vi "Stop Core.vi"(10 "final error code":i32, 11 "SinglePhotonInterferenceUI in":refnum<class "SinglePhotonInterferenceUI.lvclass">) -> (3 "SinglePhotonInterferenceUI out":refnum<class "SinglePhotonInterferenceUI.lvclass">)   [LabVIEW 2023, in "SinglePhotonInterferenceUI.lvlib" / "SinglePhotonInterferenceUI.lvclass"]
doc: "(<B>Filename</B>: Actor Framework.lvlib:Actor.lvclass:Stop Core.vi)\n\nDefines what the actor does before it stops. Use the <B>final error code</B> input to determine whether the actor shut down in response to an error.\n\nBy default, this method passes the Stop message along to all auto-stop nested actors. A descendant class may override this method to define additional behavior, such as shutting down any processes the actor initiated in its override of the Actor Core method."
uses:
  SinglePhotonInterferenceUI.lvclass
  <vilib>/ActorFramework/Actor/Actor.lvclass
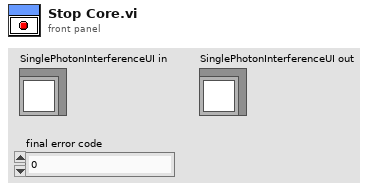
[diagram p1: front panel]
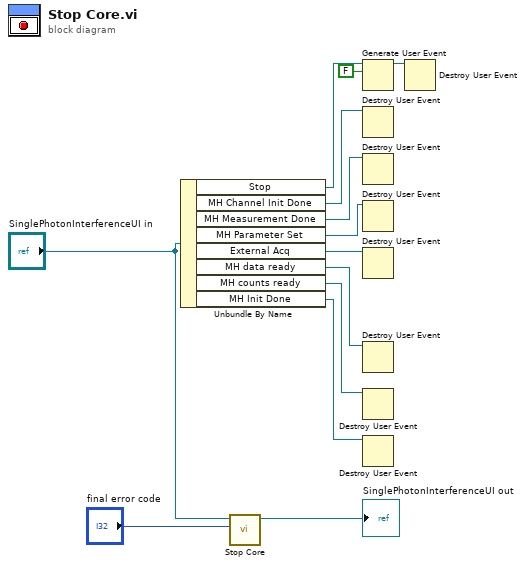
[diagram p0: block diagram]
diagram:
  n1 = Unbundle By Name("SinglePhotonInterferenceUI in") -> ("Stop"=w9:refnum<user-event>, "MH Channel Init Done"=w8:refnum<user-event>, "MH Measurement Done"=w7:refnum<user-event>, "MH Parameter Set"=w6:refnum<user-event>, "External Acq"=w5:refnum<user-event>, "MH data ready"=w4:refnum<user-event>, "MH counts ready"=w3:refnum<user-event>, "MH Init Done"=w2:refnum<user-event>)
  n2 = call-parent "Stop Core.vi"("final error code"="final error code", "Actor in"="SinglePhotonInterferenceUI in") -> ("Actor out"=→"SinglePhotonInterferenceUI out":refnum<class "SinglePhotonInterferenceUI.lvclass">)  [unwired: 9 in]
  n3 = Generate User Event(user event=w9, event data cluster=FALSE ("event data")) -> (user event out=w11:refnum<user-event>)  [unwired: 2 in, 1 out]
  n4 = Destroy User Event(user event=w8) -> ()  [unwired: 1 in, 1 out]
  n5 = Destroy User Event(user event=w7) -> ()  [unwired: 1 in, 1 out]
  n6 = Destroy User Event(user event=w6) -> ()  [unwired: 1 in, 1 out]
  n7 = Destroy User Event(user event=w5) -> ()  [unwired: 1 in, 1 out]
  n8 = Destroy User Event(user event=w4) -> ()  [unwired: 1 in, 1 out]
  n9 = Destroy User Event(user event=w3) -> ()  [unwired: 1 in, 1 out]
  n10 = Destroy User Event(user event=w2) -> ()  [unwired: 1 in, 1 out]
  n11 = Destroy User Event(user event=w11) -> ()  [unwired: 1 in, 1 out]
